vi "Anritsu VNA Read Channel.vi"(7 "Anritsu VNA":T1, 8 "error in (no error)":errorcluster, 11 "VISA Resource Name":refnum<visa-resource-name>) -> (0 "error out":errorcluster, 2 "Channel":i8, 3 "dup VISA Resource Name":refnum<visa-resource-name>)   [LabVIEW 2011]
doc: "This VI for the HP 8753B is used to read the number of stimulus points."
uses:
  TypeDefs/Anritsu VNA Instrument Info.ctl
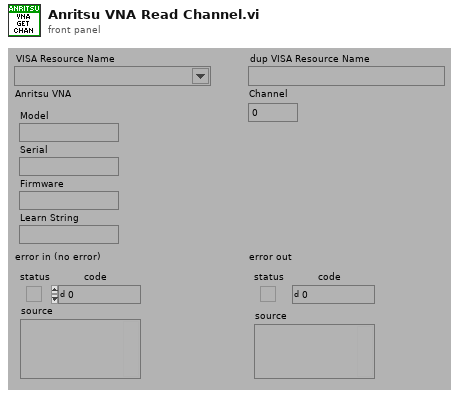
[diagram p1: front panel]
types:
  T1 = typedef "Anritsu VNA Instrument Info.ctl" = cluster{"Model":string, "Serial":string, "Firmware":string, "Learn String":string}
  T2 = typedef "Anritsu VNA Model.ctl" = enum16{"Not Supported", "37XXXX", "MS20XXX", "MS462XX", "MS464XX"}
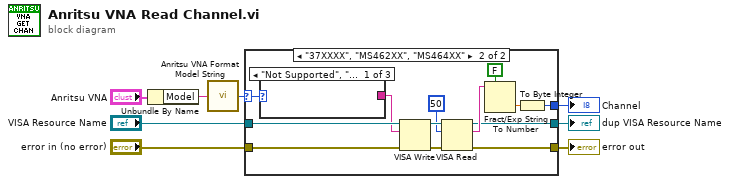
[diagram p0: block diagram]
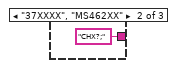
[diagram p3: hidden frame]
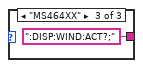
[diagram p4: hidden frame]
diagram:
  n1 = Unbundle By Name("Anritsu VNA") -> ("Model"=w2:string)
  n2 = call "Anritsu VNA Format Model String.vi"("Model"=w2) -> ("Model"=w1:T2)
  n3 = case shown="\"37XXXX\", \"MS462XX\", \"MS464XX\"" w1 {
    selector: w1 -> [_ w11]
    tunnel: [w10 w20] -> w8
    tunnel: [w9 w19] -> w7
    tunnel: "VISA Resource Name" -> [w10 w18]
    tunnel: "error in (no error)" -> [w9 w17]
    tunnel: [_ w16] -> w4
    frame "Not Supported", "MS20XXX" {
      # "these VNAs don't have multiple channels."
    }
    frame "37XXXX", "MS462XX", "MS464XX" {
      n4 = case shown="\"Not Supported\", \"MS20XXX\"" w11 {
        tunnel: [_ "CHX?;" ":DISP:WIND:ACT?;"] -> w12
        frame "Not Supported", "MS20XXX" {
        }
        frame "37XXXX", "MS462XX" {
        }
        frame "MS464XX" {
        }
      }
      n5 = VISA Write(VISA resource name=w18, write buffer=w12, error in (no error)=w17) -> (VISA resource name out=w15:refnum<visa-resource-name>, error out=w23:errorcluster)  [unwired: 1 out]
      n6 = VISA Read(VISA resource name=w15, byte count=u32 50, error in (no error)=w23) -> (VISA resource name out=w20:refnum<visa-resource-name>, read buffer=w22:string, error out=w19:errorcluster)  [unwired: 1 out]
      n7 = Fract/Exp String To Number(use system decimal point (T)=FALSE, string=w22) -> (number=w21:dbl)  [unwired: 3 out]
      n8 = To Byte Integer(number=w21) -> (8bit integer=w16:i8)
    }
  }
  "Channel" <- w4
  "dup VISA Resource Name" <- w8
  "error out" <- w7
